vi "main screen V2_Backup.vi"() -> ()   [LabVIEW 2020]
uses:
  <vilib>/DAQmx/read.llb/DAQmx Read (Analog 1D DBL NChan 1Samp).vi
  <vilib>/DAQmx/miscellaneous.llb/DAQmx Fill In Error Info.vi
  <vilib>/Utility/file.llb/Write Delimited Spreadsheet (string).vi
  <vilib>/Utility/file.llb/Write Delimited Spreadsheet (DBL).vi
  <vilib>/vision/driver/NI_Vision_Acquisition_Software.lvlib
panel:
  in  "physical channels 2":tag="cDAQ1Mod1/ai1,cDAQ1Mod1/ai2"
  out "Saving Data":bool
  out "System Time":dbl
  in  "Sample Rate":dbl=90.0
  out "error out 2":errorcluster
  out "Image 2":T1(plugin-control)
  out "Image":T1(plugin-control)
  out "error out":errorcluster
  out "Clock":dbl[](graph)
  out "T.C 2":dbl[](graph)
  out "T.C 3":dbl[](graph)
  out "T.C 4":dbl[](graph)
  out "T.C 5":dbl[](graph)
  out "T.C 6":dbl[](graph)
  out "T.C 7":dbl[](graph)
  out "Front Diode":dbl[](graph)
  out "Rear Diode":dbl[](graph)
  out "T.C 1":dbl[](graph)
  out "T.C 8":dbl[](graph)
  in  "stop":bool
  in  "TC channel":tag="cDAQ1Mod3/ai0,cDAQ1Mod3/ai1,cDAQ1Mod3/ai2,cDAQ1Mod3/ai3,cDAQ1Mod3/ai4,cDAQ1Mod3/ai5,cDAQ1Mod3/ai6,cDAQ1Mod3/ai7"
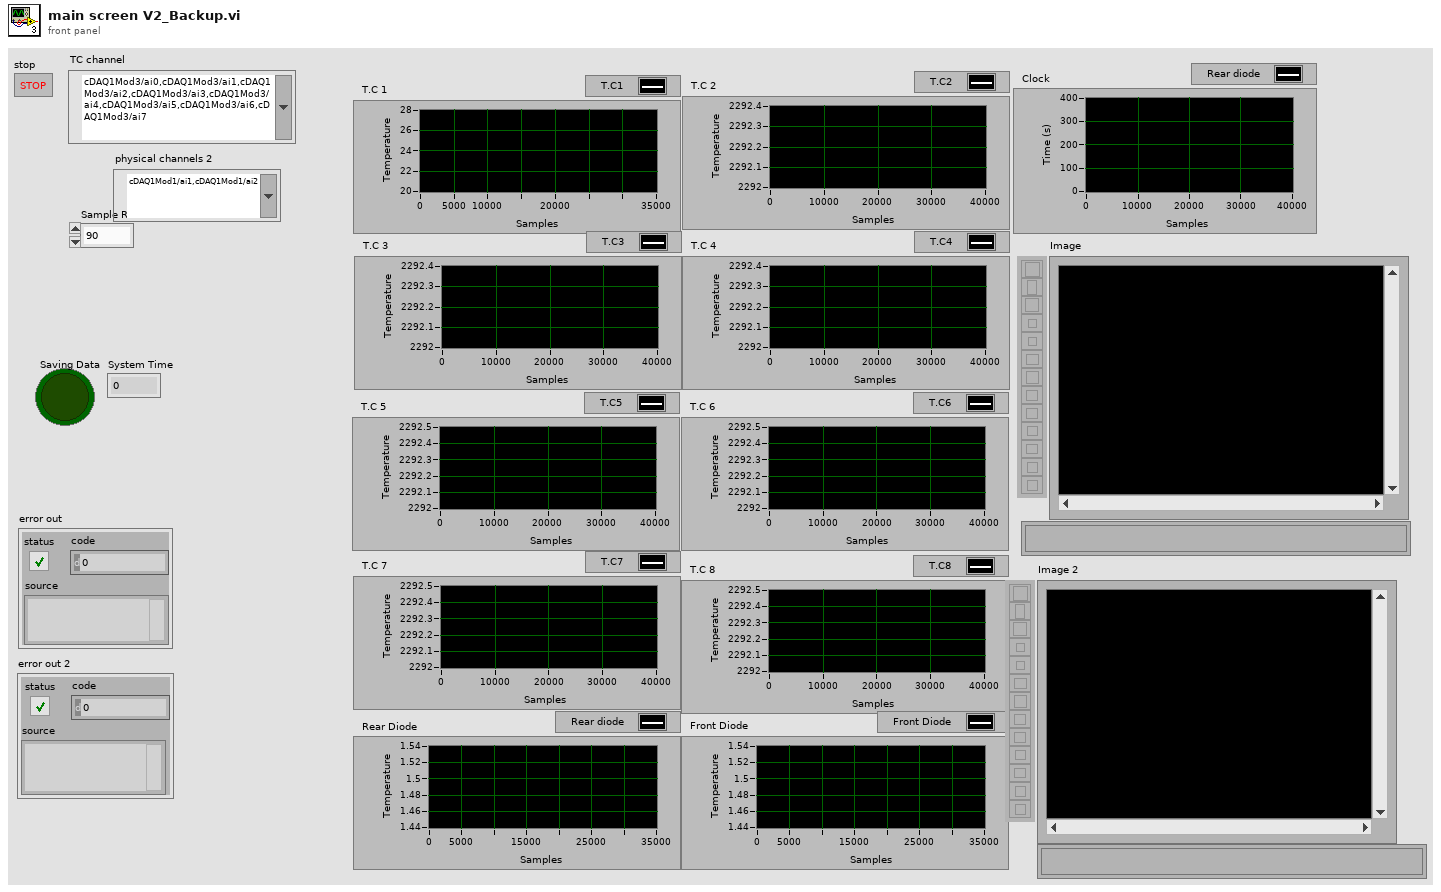
[diagram p1: front panel]
types:
  T1 = typedef "IMAQ Image.ctl" = refnum<image>
  T2 = typedef "IMAQdx.ctl" = refnum<k21>
  T3 = typedef "IMAQ AVI2 Refnum.ctl" = refnum<k20>
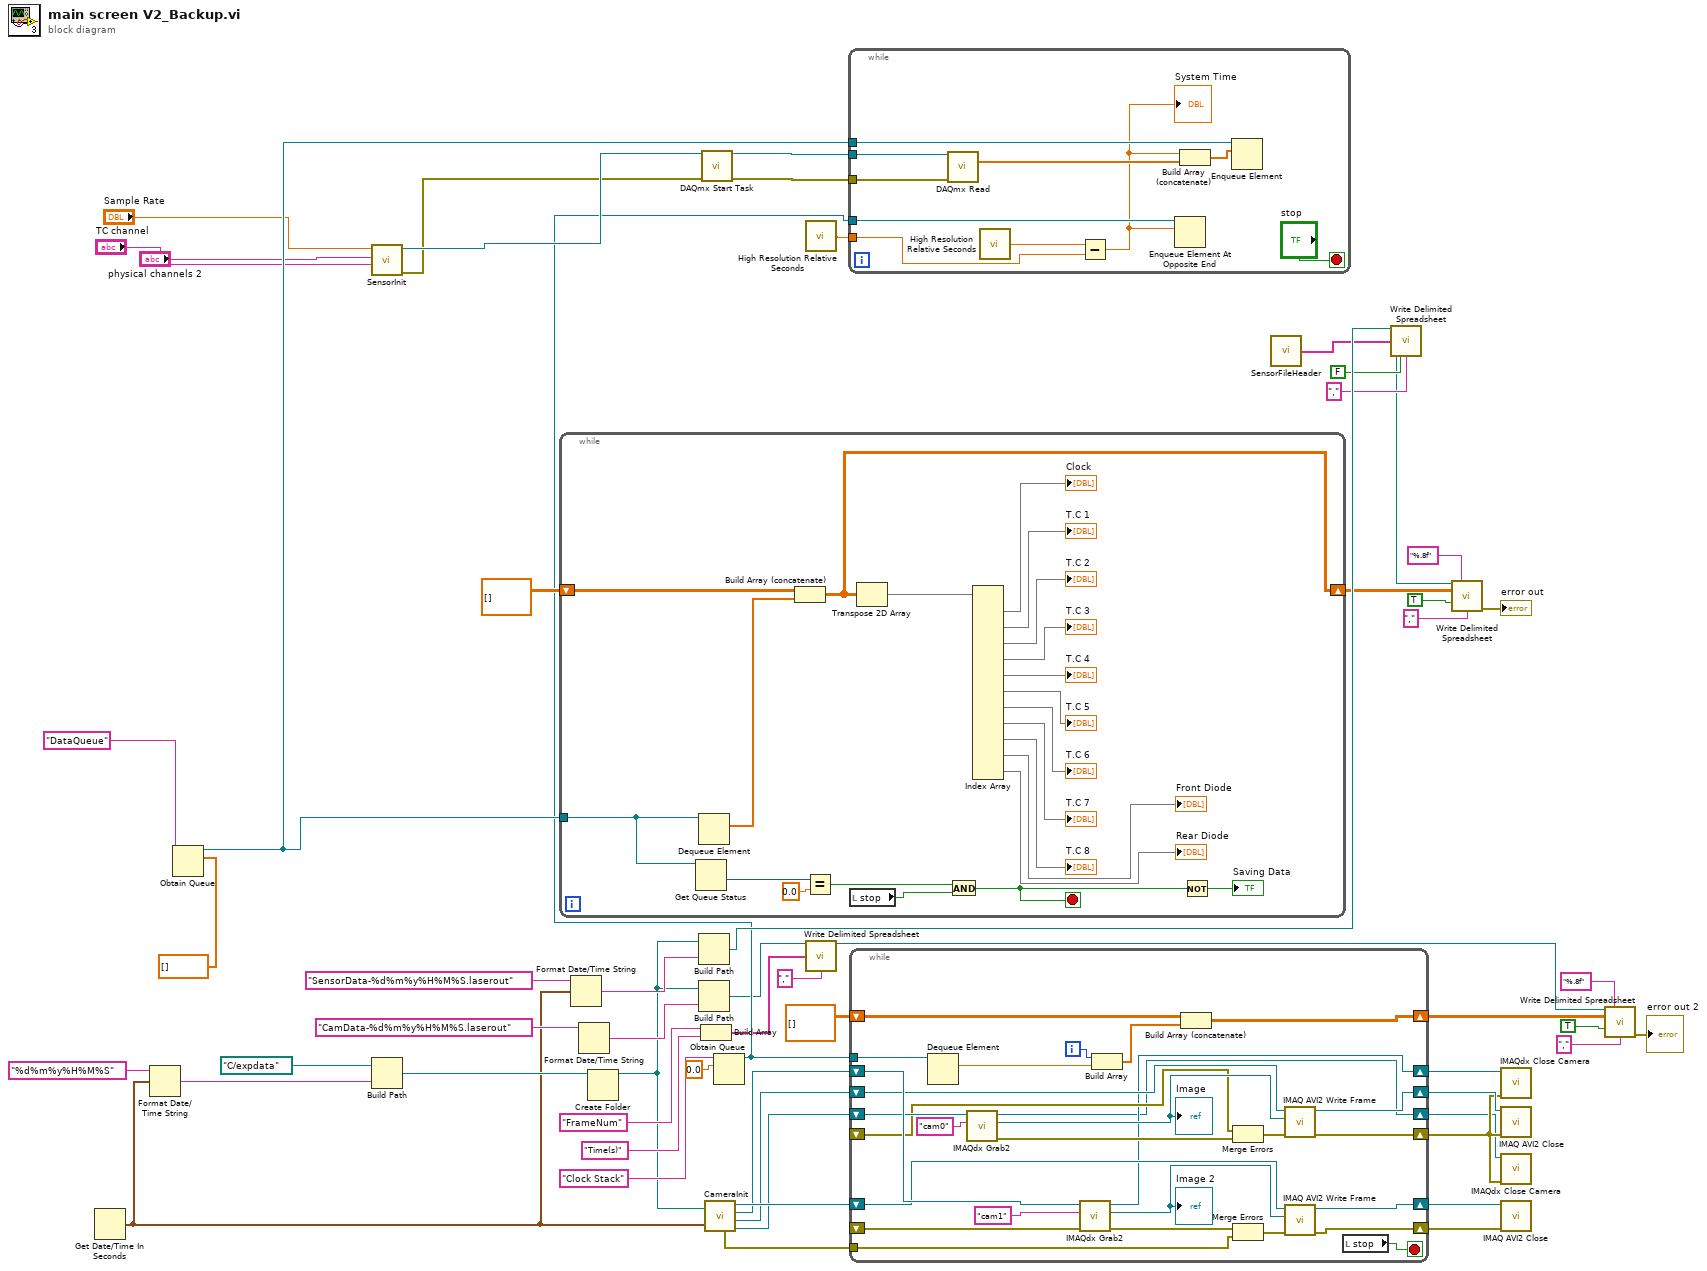
[diagram p0: block diagram]
diagram:
  n1 = Get Date/Time In Seconds() -> (seconds since 1Jan1904=w3:timestamp)
  n2 = Format Date/Time String(time format string (%c)="%d%m%y%H%M%S", seconds (now)=w3) -> (date/time string=w46:string)  [unwired: 1 in]
  n3 = Obtain Queue(name (unnamed)="DataQueue", element data type=dbl[] []) -> (queue out=w58:refnum<queue>)  [unwired: 3 in, 2 out]
  n4 = call "SensorInit.vi"("TC channel"="TC channel", "physical channels in"="physical channels 2", "Sample Rate"="Sample Rate") -> ("error out"=w51:errorcluster, "Task out"=w53:refnum<k21>)  [unwired: 7 in]
  n5 = Build Path(base path=path "C:/expdata", name or relative path=w46) -> (appended path=w45:path)
  n6 = while {
    tunnel: w58 -> [w63]
    shift-right: [w67] -> w36
    shift-left: dbl[][] [] -> [w80]
    stop <- w60 stop-if-true
    n7 = Get Queue Status(queue=w63) -> (# pending insert=w62:i32)  [unwired: 2 in, 7 out]
    n8 = Dequeue Element(queue=w63) -> (element=w79:dbl[])  [unwired: 2 in, 3 out]
    n9 = Build Array (concatenate)(w80, w79) -> (w67:dbl[][])
    n10 = Equal?(x=w62, y=0.0) -> (x = y?=w65:bool)
    n11 = local read "stop"() -> (w61:bool)
    n12 = Transpose 2D Array(2D array=w67) -> (transposed array=w66:dbl[][])
    n13 = And(x=w65, y=w61) -> (x .and. y?=w60:bool)
    n14 = Index Array(array=w66) -> (element #1=→"Clock":dbl[], element #2=→"T.C 1":dbl[], element #3=→"T.C 2":dbl[], element #4=→"T.C 3":dbl[], element #5=→"T.C 4":dbl[], element #6=→"T.C 5":dbl[], element #7=→"T.C 6":dbl[], element #8=→"T.C 7":dbl[], element #9=→"T.C 8":dbl[], element #10=→"Front Diode":dbl[], element #11=→"Rear Diode":dbl[])  [unwired: 22 in]
    n15 = Not(x=w60) -> (.not. x?=→"Saving Data":bool)
  }
  n16 = Format Date/Time String(time format string (%c)="SensorData-%d%m%y%H%M%S.laserout", seconds (now)=w3) -> (date/time string=w43:string)  [unwired: 1 in]
  n17 = Format Date/Time String(time format string (%c)="CamData-%d%m%y%H%M%S.laserout") -> (date/time string=w24:string)  [unwired: 2 in]
  n18 = Create Folder(path (use dialog)=w45) -> (created path=w2:path)  [unwired: 2 in, 2 out]
  n19 = Build Path(base path=w2, name or relative path=w43) -> (appended path=w42:path)
  n20 = Build Path(base path=w2, name or relative path=w24) -> (appended path=w23:path)
  n21 = Build Array("FrameNum", "Time(s)") -> (w19:string[])
  n22 = call <vilib>:"DAQmx Start Task.vi"("task/channels in"=w53, "error in"=w51) -> ("task out"=w52:refnum<k21>, "error out"=w50:errorcluster)  [unwired: 12 in]
  n23 = call "CameraInit.vi"("start time"=w3, "folder path"=w2) -> ("BW Session Out"=w4:T2, "BW AVI out"=w5:T3, "Color session out"=w6:T2, "Color AVI out"=w7:T3, "error out"=w1:errorcluster)
  n24 = Obtain Queue(name (unnamed)="Clock Stack", element data type=0.0) -> (queue out=w26:refnum<queue>)  [unwired: 3 in, 2 out]
  n25 = call <vilib>:"High Resolution Relative Seconds.vi"() -> ("relative seconds"=w54:dbl)
  n26 = call-poly <vilib>:"Write Delimited Spreadsheet.vi"("file path (dialog if empty)"=w23, "1D data"=w19, "delimiter (\\t)"="," ("delimiter (\\t)")) -> ("new file path (Not A Path if cancelled)"=w15:path)  [unwired: 11 in, 1 out]
  n27 = while {
    tunnel: w58 -> [w90]
    tunnel: w52 -> [w89]
    tunnel: w50 -> [w88]
    tunnel: w54 -> [w87]
    tunnel: w26 -> [w82]
    stop <- "stop" stop-if-true
    n28 = call-poly <vilib>:"DAQmx Read.vi"("task/channels in"=w89, "error in"=w88) -> ("data"=w85:dbl[])  [unwired: 11 in, 2 out]
    n29 = call <vilib>:"High Resolution Relative Seconds.vi"() -> ("relative seconds"=w86:dbl)
    n30 = Subtract(x=w86, y=w87) -> (x-y=w81:dbl)
    "System Time" <- w81
    n31 = Enqueue Element At Opposite End(queue=w82, element=w81) -> ()  [unwired: 2 in, 3 out]
    n32 = Build Array (concatenate)(w81, w85) -> (w84:dbl[])
    n33 = Enqueue Element(queue=w90, element=w84) -> ()  [unwired: 2 in, 3 out]
  }
  n34 = while {
    shift-right: [w102] -> w29
    shift-left: w6 -> [w116]
    shift-right: [w104] -> w31
    shift-left: _ -> [w115]
    shift-right: [w106] -> w33
    shift-left: w7 -> [w114]
    shift-right: [w101] -> w28
    shift-left: w4 -> [w111]
    shift-right: [w105] -> w32
    shift-left: w5 -> [w110]
    shift-right: [w103] -> w30
    shift-left: _ -> [w108]
    tunnel: w26 -> [w100]
    shift-right: [w97] -> w14
    shift-left: dbl[][] [] -> [w98]
    tunnel: w1 -> [w91]
    i -> [w95]
    stop <- w96 stop-if-true
    n35 = Dequeue Element(queue=w100) -> (element=w94:dbl)  [unwired: 2 in, 3 out]
    n36 = call <vilib>:"IMAQdx Grab2.vi"("Image In"="cam0" ("Image Name"), "Session In"=w111) -> ("error out"=w109:errorcluster, "Image Out"=w118:T1, "Session Out"=w101:T2)  [unwired: 6 in, 1 out]
    "Image" <- w118
    n37 = call <vilib>:"IMAQdx Grab2.vi"("error in"=w115, "Image In"="cam1" ("Image Name"), "Session In"=w116) -> ("error out"=w112:errorcluster, "Image Out"=w117:T1, "Session Out"=w102:T2)  [unwired: 5 in, 1 out]
    "Image 2" <- w117
    n38 = Build Array(w95, w94) -> (w99:dbl[])
    n39 = Build Array (concatenate)(w98, w99) -> (w97:dbl[][])
    n40 = Merge Errors(w108, w109) -> (w107:errorcluster)
    n41 = Merge Errors(w112, w91) -> (w113:errorcluster)
    n42 = call "IMAQ AVI2 Write Frame"("error in (no error)"=w107, "Image"=w118, "AVI Refnum"=w110) -> ("error out"=w103:errorcluster, "AVI Refnum (duplicate)"=w105:T3)  [unwired: 6 in, 1 out]
    n43 = call "IMAQ AVI2 Write Frame"("error in (no error)"=w113, "Image"=w117, "AVI Refnum"=w114) -> ("error out"=w104:errorcluster, "AVI Refnum (duplicate)"=w106:T3)  [unwired: 6 in, 1 out]
    n44 = local read "stop"() -> (w96:bool)
  }
  n45 = call "SensorFileHeader.vi"() -> ("Header\nOut"=w41:string[])
  n46 = call-poly <vilib>:"Write Delimited Spreadsheet.vi"("file path (dialog if empty)"=w42, "1D data"=w41, "transpose? (no:F)"=FALSE, "delimiter (\\t)"="," ("delimiter (\\t)")) -> ("new file path (Not A Path if cancelled)"=w35:path)  [unwired: 10 in, 1 out]
  n47 = call-poly <vilib>:"Write Delimited Spreadsheet.vi"("file path (dialog if empty)"=w35, "format (%.3f)"="%.8f", "2D data"=w36, "append to file? (new file:F)"=TRUE, "delimiter (\\t)"="," ("delimiter (\\t)")) -> ("error out"=→"error out":errorcluster)  [unwired: 9 in, 1 out]
  n48 = call <vilib>:"IMAQdx Close Camera.vi"("error in"=w30, "Session In"=w29) -> ()  [unwired: 9 in, 1 out]
  n49 = call "IMAQ AVI2 Close"("error in (no error)"=w30, "AVI Refnum"=w32) -> ()  [unwired: 9 in, 1 out]
  n50 = call <vilib>:"IMAQdx Close Camera.vi"("error in"=w30, "Session In"=w28) -> ()  [unwired: 9 in, 1 out]
  n51 = call "IMAQ AVI2 Close"("error in (no error)"=w31, "AVI Refnum"=w33) -> ()  [unwired: 9 in, 1 out]
  n52 = call-poly <vilib>:"Write Delimited Spreadsheet.vi"("file path (dialog if empty)"=w15, "format (%.3f)"="%.8f", "2D data"=w14, "append to file? (new file:F)"=TRUE, "delimiter (\\t)"="," ("delimiter (\\t)")) -> ("error out"=→"error out 2":errorcluster)  [unwired: 9 in, 1 out]
